vi "AndorAdjustHistogram.vi"(8 "error in (no error)":errorcluster, 11 "Original Image":T1(plugin-control)) -> (0 "error out":errorcluster, 1 "MaxValue":dbl, 2 "MinValue":dbl, 3 "Processed Image":T1(plugin-control))   [LabVIEW 2018, in "AndorOWN.lvlib"]
uses:
  AndorOWN.lvlib
  <vilib>/vision/NI_Vision_Development_Module.lvlib
  <resource>/objmgr/IMAQImage.rc
panel:
  in  "Stop":bool
  out "Histogram":T2(graph)={"Starting Value"=0.0, "Incremental Value"=0.5, "Histogram"=array[65536 elements]}
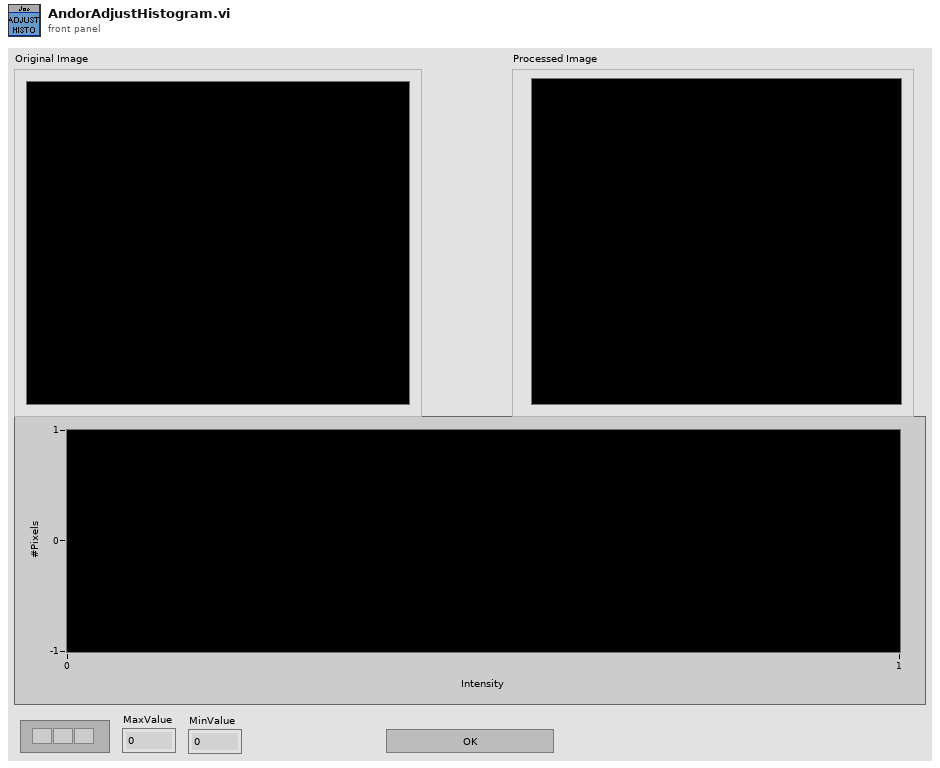
[diagram p1: front panel]
types:
  T1 = typedef "IMAQ Image.ctl" = refnum<image>
  T2 = cluster{"Starting Value":sgl, "Incremental Value":sgl, "Histogram":u32[]}
  T3 = typedef "LVCursorListTypeDef.ctl" = cluster{"Name":string, "Color":u32, "Style":u8, "Point Style":u8, "Name Visible":bool, "Allow Drag":bool, "Cursor Mode":u32, "Plot":i32, "Index":i32, "Position":cluster{"X":dbl, "Y":dbl}, "X Scale":u32, "Y Scale":u32, "Watch Plots":i32[], "Watch All Plots":bool, "Plot Area":i32, "Label Offset":cluster{"X":dbl, "Y":dbl}}[]
  T4 = cluster{"Name":string, "Color":u32, "Style":u8, "Point Style":u8, "Name Visible":bool, "Allow Drag":bool, "Cursor Mode":u32, "Plot":i32, "Index":i32, "Position":cluster{"X":dbl, "Y":dbl}, "X Scale":u32, "Y Scale":u32, "Watch Plots":i32[], "Watch All Plots":bool, "Plot Area":i32, "Label Offset":cluster{"X":dbl, "Y":dbl}}
  T5 = cluster{"Name":string, "Color":u32, "Style":u8, "Point Style":u8, "Name Visible":bool, "Allow Drag":bool, "Cursor Mode":u32, "Plot":i32, "Index":i32, "Position":cluster{"X":dbl, "Y":dbl}, "X Scale":u32, "Y Scale":u32, "Watch Plots":i32[], "Watch All Plots":bool, "Plot Area":i32, "Label Offset":cluster{"X":dbl, "Y":dbl}}[]
  T6 = enum32{"Linear", "Log", "Exp", "Square", "Square root", "Power X", "Power 1/X"}
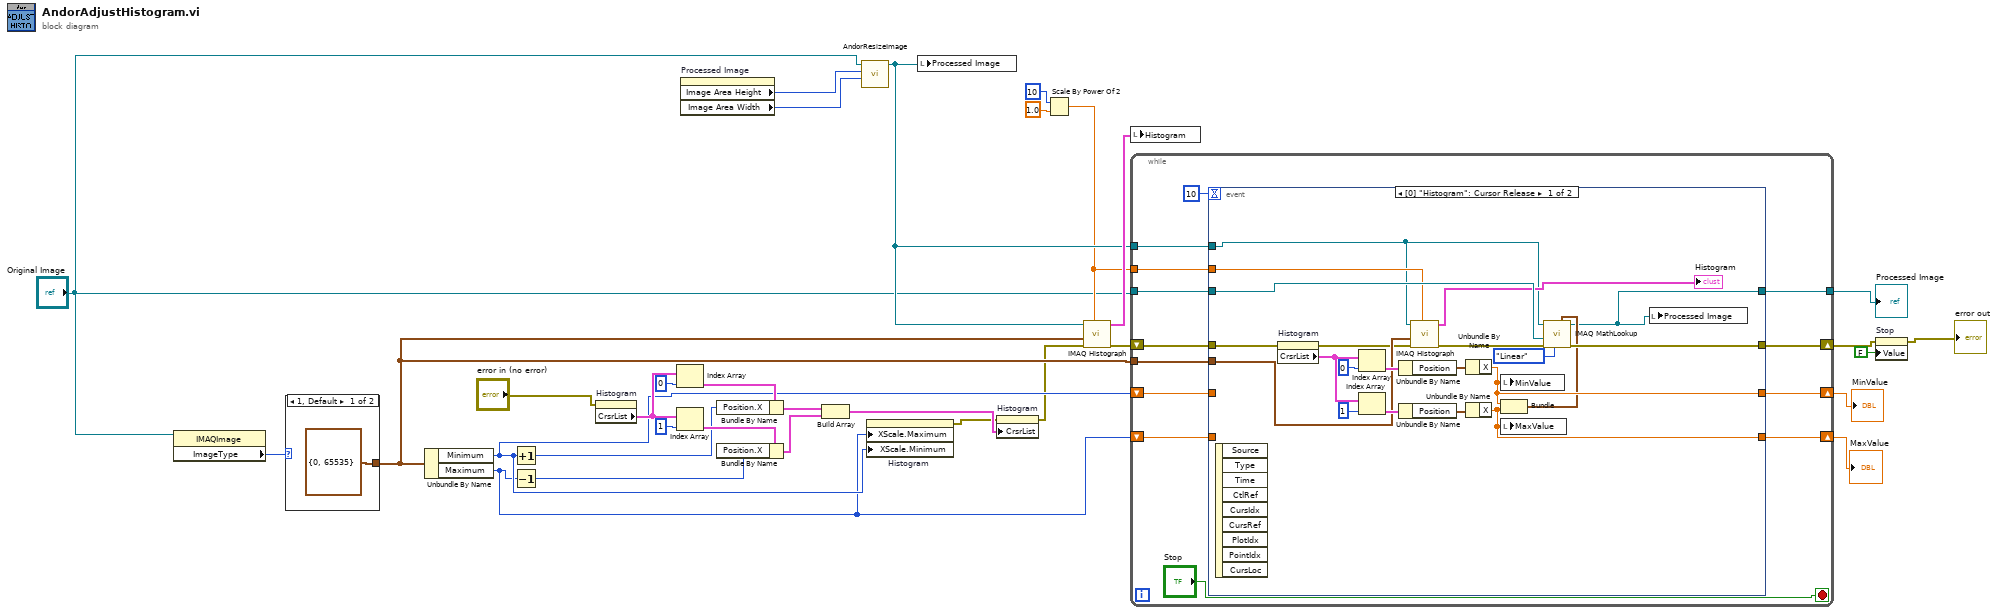
[diagram p0: block diagram]
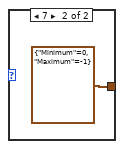
[diagram p2: hidden frame]
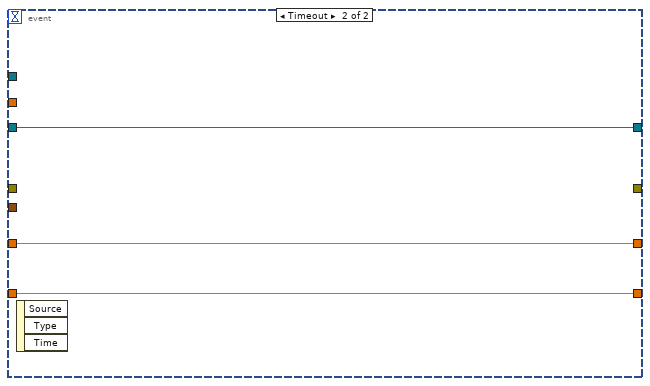
[diagram p3: hidden frame]
diagram:
  n1 = property class="IMAQImage"(reference="Original Image") -> ("ImageType"=w2:u32)  [unwired: 1 in, 2 out]
  n2 = case shown="1, Default" w2 {
    tunnel: [cluster{"Minimum":u16, "Maximum":u16} {"Minimum"=0, "Maximum"=65535} ("Interval Range") cluster{"Minimum":i16, "Maximum":i16} {"Minimum"=0, "Maximum"=-1} ("Interval Range")] -> w30
    frame 1, Default {
    }
    frame 7 {
    }
  }
  n3 = Unbundle By Name(w30) -> ("Minimum"=w19:u16, "Maximum"=w18:u16)
  n4 = Increment(x=w19) -> (x+1=w14:u16)
  n5 = Decrement(x=w18) -> (x-1=w13:u16)
  n6 = property on="Histogram" class="WFGraph (strict)"(error in="error in (no error)") -> ("CrsrList"=w24:T3)  [unwired: 1 in, 2 out]
  n7 = Index Array(array=w24, index=0) -> (element=w23:T4)
  n8 = Index Array(array=w24, index=1) -> (element=w22:T4)
  n9 = property on="Processed Image" class="ImageControl"() -> ("Image Area Height"=w17:u32, "Image Area Width"=w16:u32)  [unwired: 2 in, 2 out]
  n10 = Bundle By Name(cluster=w23, "Position.X"=w14) -> (w20:T4)
  n11 = Bundle By Name(cluster=w22, "Position.X"=w13) -> (w21:T4)
  n12 = Build Array(w20, w21) -> (w12:T5)
  n13 = call "AndorResizeImage.vi"("Image Area Width"=w16, "Image Area Height"=w17, "Refnum in"="Original Image") -> ("Refnum out"=w9:T1)  [unwired: 7 in, 1 out]
  n14 = property on="Histogram" class="WFGraph (strict)"("XScale.Maximum"=w18, "XScale.Minimum"=w19) -> (error out=w11:errorcluster)  [unwired: 2 in, 1 out]
  n15 = local write "Processed Image"(w9) -> ()
  n16 = property on="Histogram" class="WFGraph (strict)"(error in=w11, "CrsrList"=w12) -> (error out=w10:errorcluster)  [unwired: 1 in, 1 out]
  n17 = Scale By Power Of 2(n=i16 10, x=1.0) -> (x*2^n=w8:dbl)
  n18 = call "IMAQ Histograph"("Number of Classes"=w8, "error in (no error)"=w10, "Interval Range"=w30, "Image"=w9) -> ("error out"=w15:errorcluster, "Histogram Graph"=w28:T2)  [unwired: 4 in, 2 out]
  n19 = local write "Histogram"(w28) -> ()
  n20 = while {
    shift-right: [w42] -> w32
    shift-left: w18 -> [w40]
    shift-right: [w41] -> w31
    shift-left: w19 -> [w39]
    tunnel: w30 -> [w38]
    shift-right: [w37] -> w6
    shift-left: w15 -> [w36]
    tunnel: w9 -> [w47]
    tunnel: "Original Image" -> [w44]
    tunnel: [w43] -> w3
    tunnel: w8 -> [w35]
    stop <- "Stop" stop-if-true
    n21 = event shown="[0] \"Histogram\": Cursor Release" {
      selector: _ -> [_ _]
      dyn-events: _ -> [_ _]
      timeout: 10 -> [_ _]
      tunnel: w47 -> [w51 _]
      tunnel: w44 -> [w60 w69]
      tunnel: [w48 w69] -> w43
      tunnel: [w55 w70] -> w42
      tunnel: [w56 w71] -> w41
      tunnel: w40 -> [_ w70]
      tunnel: w39 -> [_ w71]
      tunnel: w38 -> [w61 _]
      tunnel: [w54 _] -> w37
      tunnel: w36 -> [w58 _]
      tunnel: w35 -> [w52 _]
      event "Histogram": Cursor Release {
        n22 = event-data() -> ()  [unwired: 1 in, 9 out]
        n23 = property on="Histogram" class="WFGraph (strict)"(error in=w58) -> (error out=w57:errorcluster, "CrsrList"=w66:T3)  [unwired: 1 in, 1 out]
        n24 = Index Array(array=w66, index=0) -> (element=w63:T4)
        n25 = Index Array(array=w66, index=1) -> (element=w68:T4)
        n26 = Unbundle By Name(w63) -> ("Position"=w62:cluster{"X":dbl, "Y":dbl})
        n27 = Unbundle By Name(w68) -> ("Position"=w67:cluster{"X":dbl, "Y":dbl})
        n28 = call "IMAQ Histograph"("Number of Classes"=w52, "error in (no error)"=w57, "Interval Range"=w61, "Image"=w51) -> ("error out"=w59:errorcluster, "Histogram Graph"=→"Histogram":T2)  [unwired: 4 in, 2 out]
        n29 = Unbundle By Name(w62) -> ("X"=w56:dbl)
        n30 = Unbundle By Name(w67) -> ("X"=w55:dbl)
        n31 = local write "MinValue"(w56) -> ()
        n32 = Bundle("X"=w56, "X"=w55) -> (w49:cluster{"X":dbl, "X":dbl})  [unwired: 1 in]
        n33 = local write "MaxValue"(w55) -> ()
        n34 = call "IMAQ MathLookup"("Range"=w49, "Operator"=T6."Linear", "error in (no error)"=w59, "Image Dst"=w60, "Image Src"=w51) -> ("error out"=w54:errorcluster, "Image Dst Out"=w48:T1)  [unwired: 5 in]
        n35 = local write "Processed Image"(w48) -> ()
      }
      event Timeout {
        n36 = event-data() -> ()  [unwired: 1 in, 3 out]
      }
    }
  }
  "MaxValue" <- w32
  "MinValue" <- w31
  "Processed Image" <- w3
  n37 = property on="Stop" class="Bool (strict)"(error in=w6, "Value"=FALSE ("Stop")) -> (error out=→"error out":errorcluster)  [unwired: 1 in, 1 out]
